vi "LS372Monitor_Standalone.vi"() -> ()   [LabVIEW 2014]
uses:
  Instrument_Setup.vi
  Global/Global Variables/Data_Display_global.vi
panel:
  in  "Stopp":bool
  out "Temperatures":cluster{timestamp[], dbl[]}[](graph)
  out "Analog Power":cluster{timestamp[], dbl[]}[](graph)
  out "Heater Power":cluster{timestamp[], dbl[]}(graph)
  in  "Update Lakeshore":bool
  out "MC Heater Output":dbl
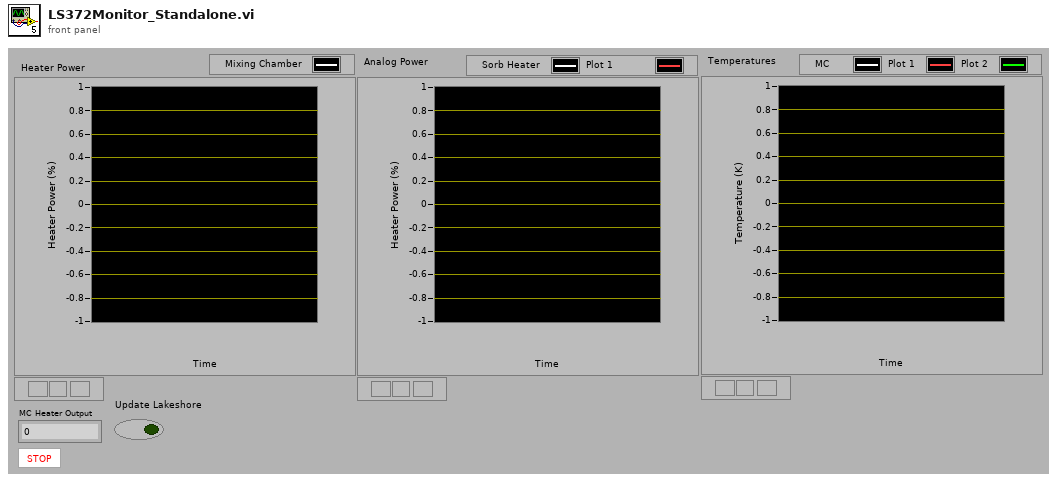
[diagram p1: front panel]
types:
  T1 = cluster{"Control Temperature":dbl[], "Still Temperature":dbl[], "Sorb Temperature":dbl[], "Time":timestamp[], "Analog Out 1 (Sorb)":dbl[], "Analog Out 2 (Still)":dbl[], "MC Heater":dbl[]}
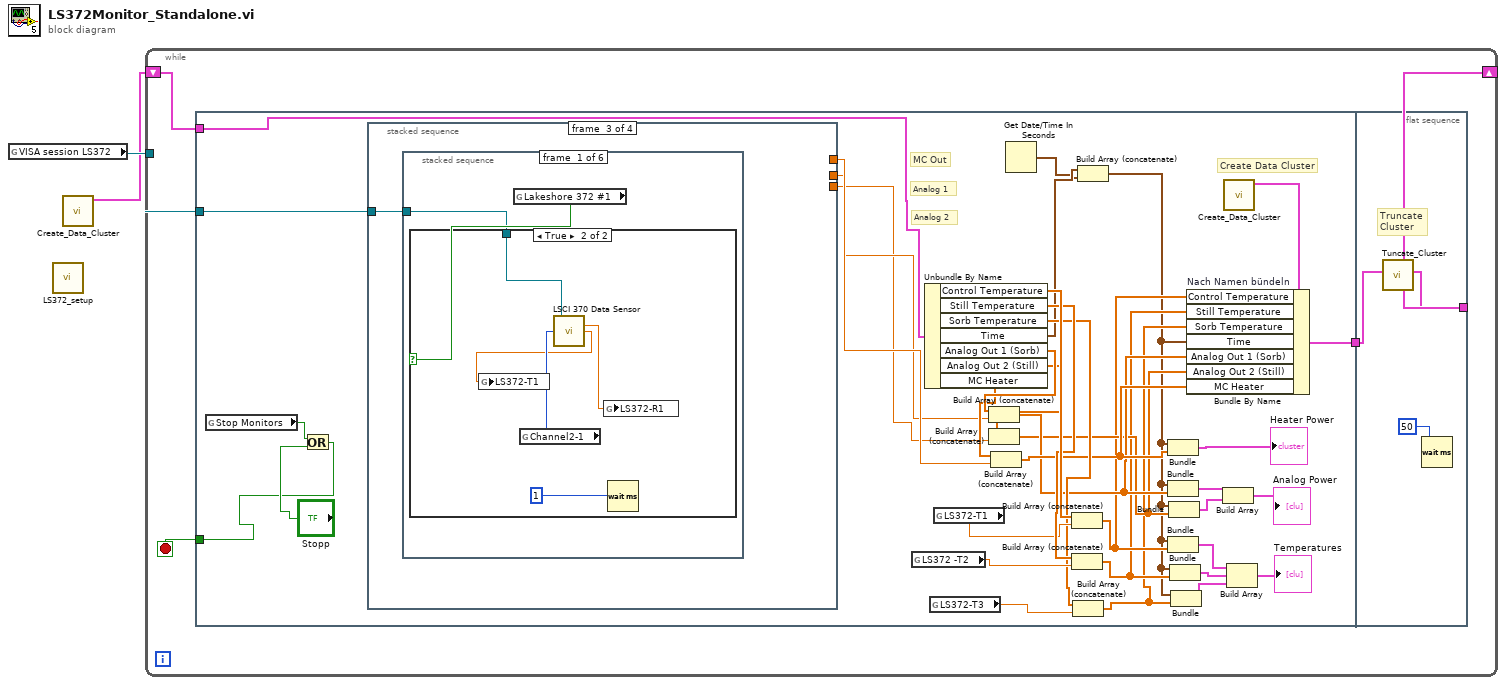
[diagram p0: block diagram]
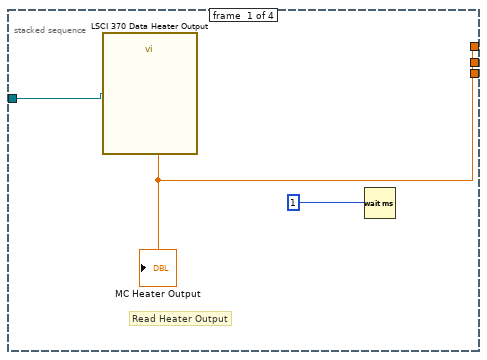
[diagram p2: hidden frame]
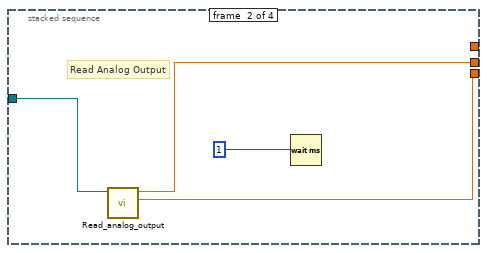
[diagram p3: hidden frame]
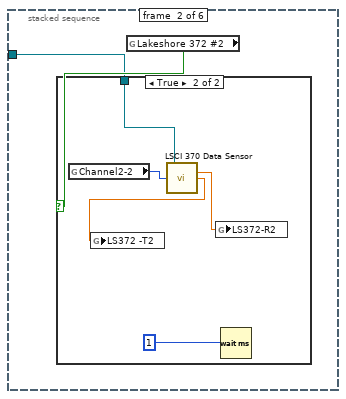
[diagram p5: hidden frame]
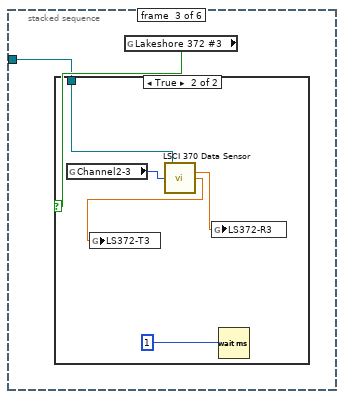
[diagram p7: hidden frame]
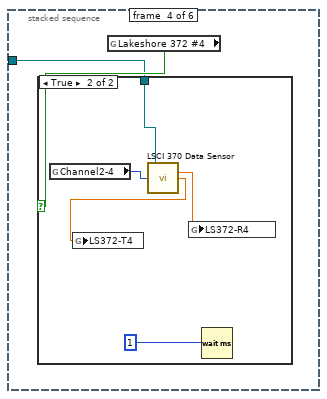
[diagram p9: hidden frame]
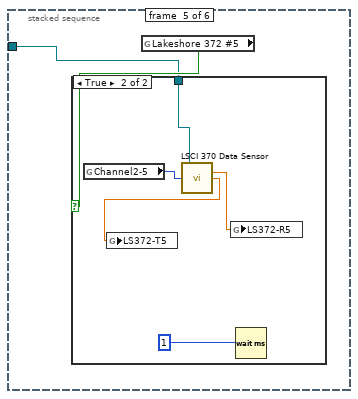
[diagram p11: hidden frame]
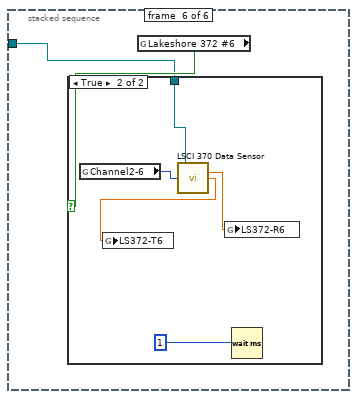
[diagram p13: hidden frame]
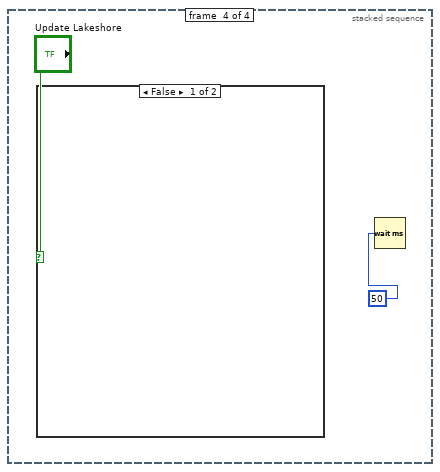
[diagram p15: hidden frame]
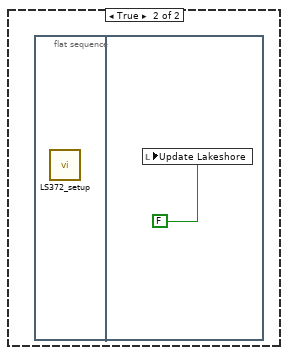
[diagram p16: hidden frame]
diagram:
  n1 = global read "Instrument_Setup.vi" "VISA session LS372"() -> (w2:refnum<visa-resource-name>)
  n2 = call "LS372_setup.vi"() -> ()  [unwired: 1 in]
  n3 = call "Create_Data_Cluster.vi"() -> ("Cluster"=w1:T1)  [unwired: 11 in]
  n4 = while {
    tunnel: w2 -> [w6]
    shift-right: [w4] -> _
    shift-left: w1 -> [w3]
    stop <- w7 stop-if-true
    n5 = flat-sequence {
      tunnel: [w8] -> w7
      tunnel: w6 -> [w43]
      tunnel: [w12] -> w5
      tunnel: w3 -> [w11]
      tunnel: w5 -> [w98]
      tunnel: [w97] -> w4
      frame #0 {
        # "Create Data Cluster"
        # "Analog 2"
        # "Analog 1"
        # "MC Out"
        n6 = global read "Data_Display_global.vi" "Stop Monitors"() -> (w10:bool)
        n7 = Or(x=w10, y="Stopp") -> (x .or. y?=w8:bool)
        n8 = stacked-sequence {
          tunnel: w43 -> [w46 w50 w51 _]
          tunnel: [w44 _ _ _] -> w15
          tunnel: [_ w48 _ _] -> w14
          tunnel: [_ w47 _ _] -> w13
          frame #0 {
            # "Read Heater Output"
            n9 = call "LSCI 370 Data Heater Output.vi"("VISA session"=w46) -> ("Heater Output"=w44:dbl)  [unwired: 12 in, 2 out]
            "MC Heater Output" <- w44
            n10 = Wait (ms)(milliseconds to wait=1) -> ()  [unwired: 1 out]
          }
          frame #1 {
            # "Read Analog Output"
            n11 = call "Read_analog_output.vi"("VISA session"=w50) -> ("Still Output"=w47:dbl, "Analog Output"=w48:dbl)  [unwired: 9 in]
            n12 = Wait (ms)(milliseconds to wait=1) -> ()  [unwired: 1 out]
          }
          frame #2 {
            n13 = stacked-sequence {
              tunnel: w51 -> [w52 w59 w66 w73 w80 w87]
              frame #0 {
                n14 = global read "Instrument_Setup.vi" "Lakeshore 372 #1"() -> (w53:bool)
                n15 = case shown="True" w53 {
                  tunnel: w52 -> [_ w54]
                  frame False {
                  }
                  frame True {
                    n16 = global read "Instrument_Setup.vi" "Channel2-1"() -> (w58:u16)
                    n17 = call "LSCI 370 Data Sensor.vi"("VISA session"=w54, "Channel (1)"=w58) -> ("Resistance Reading"=w55:dbl, "Kelvin Reading"=w56:dbl)  [unwired: 9 in, 3 out]
                    n18 = global write "Data_Display_global.vi" "LS372-T1"(w56) -> ()
                    n19 = global write "Data_Display_global.vi" "LS372-R1"(w55) -> ()
                    n20 = Wait (ms)(milliseconds to wait=1) -> ()  [unwired: 1 out]
                  }
                }
              }
              frame #1 {
                n21 = global read "Instrument_Setup.vi" "Lakeshore 372 #2"() -> (w60:bool)
                n22 = case shown="True" w60 {
                  tunnel: w59 -> [_ w63]
                  frame False {
                  }
                  frame True {
                    n23 = global read "Instrument_Setup.vi" "Channel2-2"() -> (w65:u16)
                    n24 = call "LSCI 370 Data Sensor.vi"("VISA session"=w63, "Channel (1)"=w65) -> ("Resistance Reading"=w61:dbl, "Kelvin Reading"=w62:dbl)  [unwired: 9 in, 3 out]
                    n25 = global write "Data_Display_global.vi" "LS372 -T2"(w62) -> ()
                    n26 = global write "Data_Display_global.vi" "LS372-R2"(w61) -> ()
                    n27 = Wait (ms)(milliseconds to wait=1) -> ()  [unwired: 1 out]
                  }
                }
              }
              frame #2 {
                n28 = global read "Instrument_Setup.vi" "Lakeshore 372 #3"() -> (w67:bool)
                n29 = case shown="True" w67 {
                  tunnel: w66 -> [_ w69]
                  frame False {
                  }
                  frame True {
                    n30 = global read "Instrument_Setup.vi" "Channel2-3"() -> (w72:u16)
                    n31 = call "LSCI 370 Data Sensor.vi"("VISA session"=w69, "Channel (1)"=w72) -> ("Resistance Reading"=w70:dbl, "Kelvin Reading"=w68:dbl)  [unwired: 9 in, 3 out]
                    n32 = global write "Data_Display_global.vi" "LS372-T3"(w68) -> ()
                    n33 = global write "Data_Display_global.vi" "LS372-R3"(w70) -> ()
                    n34 = Wait (ms)(milliseconds to wait=1) -> ()  [unwired: 1 out]
                  }
                }
              }
              frame #3 {
                n35 = global read "Instrument_Setup.vi" "Lakeshore 372 #4"() -> (w74:bool)
                n36 = case shown="True" w74 {
                  tunnel: w73 -> [_ w75]
                  frame False {
                  }
                  frame True {
                    n37 = global read "Instrument_Setup.vi" "Channel2-4"() -> (w79:u16)
                    n38 = call "LSCI 370 Data Sensor.vi"("VISA session"=w75, "Channel (1)"=w79) -> ("Resistance Reading"=w76:dbl, "Kelvin Reading"=w77:dbl)  [unwired: 9 in, 3 out]
                    n39 = global write "Data_Display_global.vi" "LS372-T4"(w77) -> ()
                    n40 = global write "Data_Display_global.vi" "LS372-R4"(w76) -> ()
                    n41 = Wait (ms)(milliseconds to wait=1) -> ()  [unwired: 1 out]
                  }
                }
              }
              frame #4 {
                n42 = global read "Instrument_Setup.vi" "Lakeshore 372 #5"() -> (w81:bool)
                n43 = case shown="True" w81 {
                  tunnel: w80 -> [_ w82]
                  frame False {
                  }
                  frame True {
                    n44 = global read "Instrument_Setup.vi" "Channel2-5"() -> (w86:u16)
                    n45 = call "LSCI 370 Data Sensor.vi"("VISA session"=w82, "Channel (1)"=w86) -> ("Resistance Reading"=w83:dbl, "Kelvin Reading"=w84:dbl)  [unwired: 9 in, 3 out]
                    n46 = global write "Data_Display_global.vi" "LS372-T5"(w84) -> ()
                    n47 = global write "Data_Display_global.vi" "LS372-R5"(w83) -> ()
                    n48 = Wait (ms)(milliseconds to wait=1) -> ()  [unwired: 1 out]
                  }
                }
              }
              frame #5 {
                n49 = global read "Instrument_Setup.vi" "Lakeshore 372 #6"() -> (w88:bool)
                n50 = case shown="True" w88 {
                  tunnel: w87 -> [_ w89]
                  frame False {
                  }
                  frame True {
                    n51 = global read "Instrument_Setup.vi" "Channel2-6"() -> (w93:u16)
                    n52 = call "LSCI 370 Data Sensor.vi"("VISA session"=w89, "Channel (1)"=w93) -> ("Resistance Reading"=w90:dbl, "Kelvin Reading"=w91:dbl)  [unwired: 9 in, 3 out]
                    n53 = global write "Data_Display_global.vi" "LS372-T6"(w91) -> ()
                    n54 = global write "Data_Display_global.vi" "LS372-R6"(w90) -> ()
                    n55 = Wait (ms)(milliseconds to wait=1) -> ()  [unwired: 1 out]
                  }
                }
              }
            }
          }
          frame #3 {
            n56 = case shown="False" "Update Lakeshore" {
              frame False {
              }
              frame True {
                n57 = flat-sequence {
                  frame #0 {
                    n58 = call "LS372_setup.vi"() -> ()  [unwired: 1 in]
                  }
                  frame #1 {
                    n59 = local write "Update Lakeshore"(FALSE) -> ()
                  }
                }
              }
            }
            n60 = Wait (ms)(milliseconds to wait=50) -> ()  [unwired: 1 out]
          }
        }
        n61 = global read "Data_Display_global.vi" "LS372 -T2"() -> (w38:dbl)
        n62 = Unbundle By Name(w11) -> ("Control Temperature"=w41:dbl[], "Still Temperature"=w40:dbl[], "Sorb Temperature"=w37:dbl[], "Time"=w17:timestamp[], "Analog Out 1 (Sorb)"=w31:dbl[], "Analog Out 2 (Still)"=w30:dbl[], "MC Heater"=w29:dbl[])
        n63 = global read "Data_Display_global.vi" "LS372-T3"() -> (w36:dbl)
        n64 = global read "Data_Display_global.vi" "LS372-T1"() -> (w39:dbl)
        n65 = Build Array (concatenate)(w31, w14) -> (w24:dbl[])
        n66 = Build Array (concatenate)(w30, w13) -> (w23:dbl[])
        n67 = Build Array (concatenate)(w29, w15) -> (w25:dbl[])
        n68 = Get Date/Time In Seconds() -> (seconds since 1Jan1904=w16:timestamp)
        n69 = Build Array (concatenate)(w41, w39) -> (w22:dbl[])
        n70 = Build Array (concatenate)(w40, w38) -> (w21:dbl[])
        n71 = Build Array (concatenate)(w37, w36) -> (w20:dbl[])
        n72 = Build Array (concatenate)(w17, w16) -> (w19:timestamp[])
        n73 = Bundle(w19, w25) -> (→"Heater Power":cluster{timestamp[], dbl[]})  [unwired: 1 in]
        n74 = Bundle(w19, w24) -> (w28:cluster{timestamp[], dbl[]})  [unwired: 1 in]
        n75 = Bundle(w19, w22) -> (w35:cluster{timestamp[], dbl[]})  [unwired: 1 in]
        n76 = Bundle(w19, w23) -> (w27:cluster{timestamp[], dbl[]})  [unwired: 1 in]
        n77 = Bundle(w19, w21) -> (w34:cluster{timestamp[], dbl[]})  [unwired: 1 in]
        n78 = Bundle(w19, w20) -> (w33:cluster{timestamp[], dbl[]})  [unwired: 1 in]
        n79 = Build Array(w28, w27) -> (→"Analog Power":cluster{timestamp[], dbl[]}[])
        n80 = call "Create_Data_Cluster.vi"() -> ("Cluster"=w18:T1)  [unwired: 11 in]
        n81 = Bundle By Name "Nach Namen bündeln"(cluster=w18, "Control Temperature"=w22, "Still Temperature"=w21, "Sorb Temperature"=w20, "Time"=w19, "Analog Out 1 (Sorb)"=w24, "Analog Out 2 (Still)"=w23, "MC Heater"=w25) -> (w12:T1)
        n82 = Build Array(w35, w34, w33) -> (→"Temperatures":cluster{timestamp[], dbl[]}[])
      }
      frame #1 {
        # "Truncate \nCluster"
        n83 = call "Tuncate_Cluster.vi"("Eingangscluster"=w98) -> ("Cluster"=w97:T1)  [unwired: 10 in]
        n84 = Wait (ms)(milliseconds to wait=50) -> ()  [unwired: 1 out]
      }
    }
  }
